vi "HMACSHA512.vi"(8 "error in (no error)":errorcluster, 10 "Key in":u8[](array[numeric]), 11 "Data in":u8[](array[numeric])) -> (0 "error out":errorcluster, 3 "HMACSHA512 Hash":u8[](array[numeric]))   [LabVIEW 2021, in "dotNET Crypto Hashing.lvlib"]
doc: "Generates a HMAC (SHA512) hash of the data in using the provided key."
uses:
  dotNET Crypto Hashing.lvlib
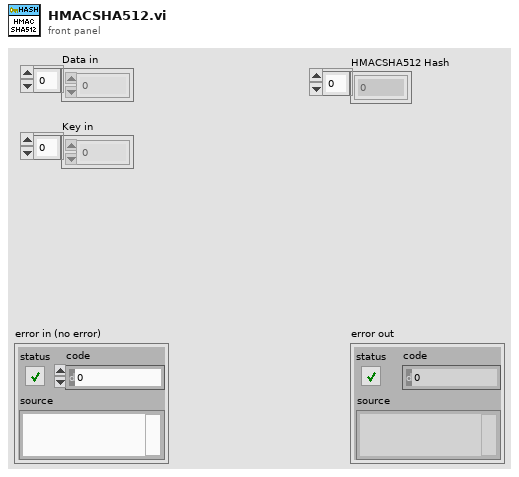
[diagram p1: front panel]
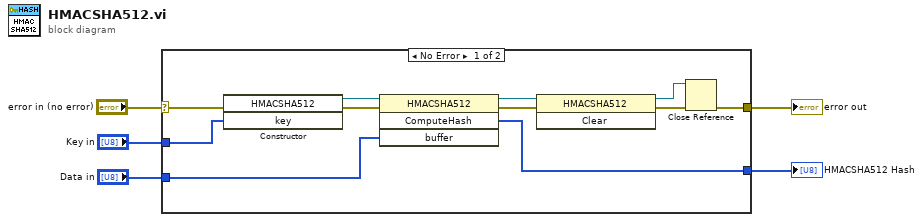
[diagram p0: block diagram]
diagram:
  n1 = case shown="No Error" "error in (no error)" {
    selector: "error in (no error)" -> [w10 w17]
    tunnel: [w9 w17] -> w4
    tunnel: [w8 _] -> w3
    tunnel: "Key in" -> [w7 _]
    tunnel: "Data in" -> [w6 _]
    frame No Error {
      n2 = constructor class="HMACSHA512"(error in=w10, "key"=w7) -> (reference out=w15:refnum<k24>, error out=w16:errorcluster)  [unwired: 2 in, 2 out]
      n3 = invoke class="HMACSHA512" method="ComputeHash"(reference=w15, error in=w16, "buffer"=w6) -> (reference out=w13:refnum<k24>, error out=w14:errorcluster, "ComputeHash"=w8:u8[])  [unwired: 1 in, 1 out]
      n4 = invoke class="HMACSHA512" method="Clear"(reference=w13, error in=w14) -> (reference out=w11:refnum<k24>, error out=w12:errorcluster)  [unwired: 1 in, 1 out]
      n5 = Close Reference(reference=w11, error in (no error)=w12) -> (error out=w9:errorcluster)
    }
    frame Error {
    }
  }
  "error out" <- w4
  "HMACSHA512 Hash" <- w3
